vi "Add Sub-Entry.vi"(8 "Error In":errorcluster, 9 "OD Sub-Entry":refnum<class "OD Sub-Entry.lvclass">, 11 "reference in":refnum<class "OD Entry.lvclass">) -> (0 "Error Out":errorcluster, 3 "reference out":refnum<class "OD Entry.lvclass">)   [LabVIEW 2024, in "Electronic Datasheet.lvlib" / "OD Entry.lvclass"]
doc: "Add an existing entry as a subobject of this OD"
uses:
  OD Entry.lvclass
  OD Sub-Entry/OD Sub-Entry.lvclass
  OD Entry.lvclass/OD Entry.ctl
  D:/git/EDS-File-Viewer/Core/OD Entry/OD Entry.lvclass
  D:/git/EDS-File-Viewer/Core/OD Sub-Entry/OD Sub-Entry.lvclass
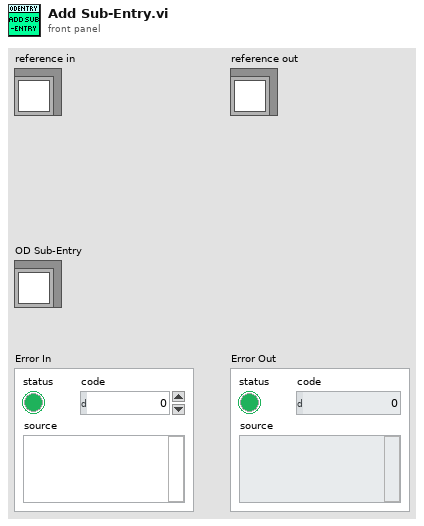
[diagram p1: front panel]
types:
  T1 = typedef "Electronic Datasheet.lvlib/OD Entry.lvclass/ObjectAttributes.ctl" = cluster{"Index":u16, "ObjectType":refnum<class "Object Type Base.lvclass">, "Denotation":string, "Count":u8, "ObjExtend":u8, "PDOtype":T2, "Label":string, "Description":string, "Sub-Entries":map{u8, refnum<class "OD Sub-Entry.lvclass">}}
  T2 = typedef "Electronic Datasheet.lvlib/PDO Mapping Type.ctl" = enum16{"NO", "OPTIONAL", "RPDO", "TPDO", "DEFAULT"}
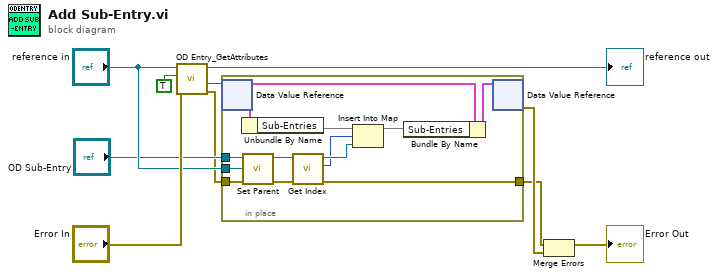
[diagram p0: block diagram]
diagram:
  n1 = call "OD Entry_GetAttributes.vi"("Error In"="Error In", "OnlyGetDvrReference(False)"=TRUE, "reference in"="reference in") -> ("Error Out"=w2:errorcluster, "DataRef"=w4:refnum<data-value>, "reference out"=→"reference out":refnum<class "OD Entry.lvclass">)  [unwired: 5 in, 1 out]
  n2 = in-place {
    in-place-border: "OD Sub-Entry" -> [w18]
    in-place-border: w2 -> [w17]
    in-place-border: [w14] -> w1
    in-place-border: "reference in" -> [w15]
    n3 = in-place-dvr #1(w4) -> (w21:T1)  [unwired: 1 out]
    n4 = Unbundle By Name(w21) -> ("Sub-Entries"=w20:map{u8, refnum<class "OD Sub-Entry.lvclass">})
    n5 = call "Set Parent.vi"("Error In"=w17, "Parent"=w15, "reference in"=w18) -> ("Error Out"=w16:errorcluster, "reference out"=w13:refnum<class "OD Sub-Entry.lvclass">)  [unwired: 7 in]
    n6 = call "Get Index.vi"("Error In"=w16, "reference in"=w13) -> ("Error Out"=w14:errorcluster, "Index"=w11:u16, "reference out"=w12:refnum<class "OD Sub-Entry.lvclass">)  [unwired: 7 in]
    n7 = Insert Into Map(map in=w20, key=w11, value=w12) -> (map out=w19:map{u8, refnum<class "OD Sub-Entry.lvclass">})  [unwired: 2 out]
    n8 = Bundle By Name(cluster=w21, "Sub-Entries"=w19) -> (w22:T1)
    n9 = in-place-dvr #1(w22) -> (w5:errorcluster)  [unwired: 1 out]
  }
  n10 = Merge Errors(w1, w5) -> (→"Error Out":errorcluster)
